vi "util_get_GPIB_address.vi"(8 "error in (no error)":errorcluster, 11 "VISA resource name":refnum<visa-resource-name>) -> (0 "error out":errorcluster, 2 "GPIB address":string, 3 "VISA resource name out":refnum<visa-resource-name>)   [LabVIEW 2016]
doc: "Determine GPIB address from VISA address."
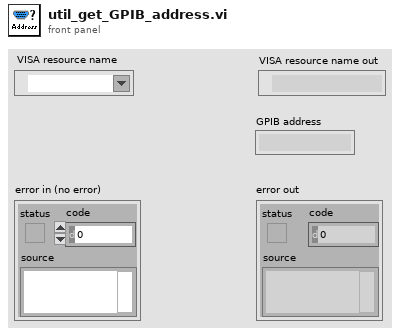
[diagram p1: front panel]
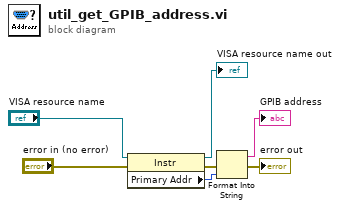
[diagram p0: block diagram]
diagram:
  n1 = property class="Instr"(reference="VISA resource name", error in="error in (no error)") -> (reference out=→"VISA resource name out":refnum<visa-resource-name>, error out=w2:errorcluster, "Primary Addr"=w5:u16)
  n2 = Format Into String(error in=w2, w5) -> (resulting string=→"GPIB address":string, error out=→"error out":errorcluster)  [unwired: 2 in]
